vi "Calculator.vi"   [LabVIEW 2016, in "Application.lvclass"]
uses:
  Application/Application.lvclass
  View/View.lvclass
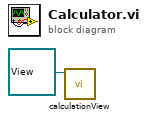
[diagram p0: block diagram]
diagram:
  n1 = call "calculationView.vi"("View.lvclass"=refnum<class "View.lvclass"> refnum) -> ()  [unwired: 11 in]
